vi "test_OneSessTwoPinOneInstrOneSiteReservation_VISAGetConnections1Pin1Connection_ReturnsOneConnection.vi"(8 "error in":errorcluster) -> (0 "error out":errorcluster, 2 "result":string, 3 "pass":bool)   [LabVIEW 2020, in "MeasurementServerTests.lvlib"]
uses:
  MeasurementServerTests.lvlib
  Runtime/MeasurementLink Session Management V1/Session Reservation/Connection.ctl
  Runtime/MeasurementLink VISA/Connection with Session.ctl
  03fc85e1-696b-4ece-a78b-f41470766ac0.vi
  54688eee-c370-47ce-a16a-9847a0fe0368.vi
  <vilib>/AdvancedString/1D String Array to Delimited String.vi
  54688eee-c370-47ce-a16a-9847a0fe0368.vi/94283ac5-2298-4b3a-b57d-7be67da3787d.vi
  54688eee-c370-47ce-a16a-9847a0fe0368.vi/f7d9c9cb-0251-4d67-81cb-70e1b0e8b69f.vi
  Runtime/MeasurementLink VISA/Get Connections - 1Pin 1Conn.vi
  <vilib>/JDP Science/JSONtext/Variant to JSON Text.vi
  <vilib>/JDP Science/JSONtext/LVClass Serializer/JSONtext LVClass Serializer.lvclass
  Runtime/MeasurementLink Session Management V1/Session Reservation/Session Reservation.lvclass
  Runtime/MeasurementLink VISA/MeasurementLink VISA.lvlib
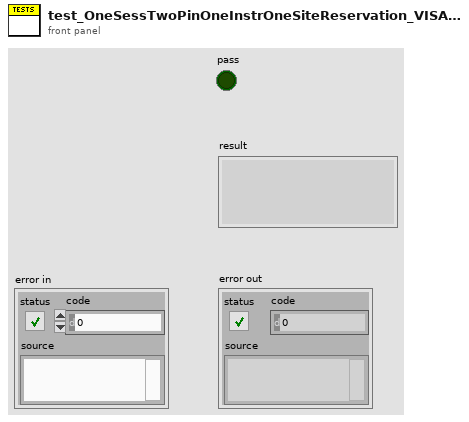
[diagram p1: front panel]
types:
  T1 = typedef "MeasurementLink VISA.lvlib/Connection with Session.ctl" = cluster{"connection":T2, "session":refnum<visa-resource-name>}
  T2 = typedef "MeasurementLink Session Management V1.lvlib/Session Reservation.lvclass/Connection.ctl" = cluster{"pin or relay name":string, "site":i32, "instrument type id":string, "channel":string}
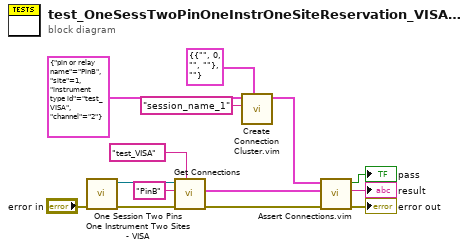
[diagram p0: block diagram]
diagram:
  n1 = call "One Session Two Pins One Instrument Two Sites - VISA.vi"("error in"="error in") -> ("error out"=w4:errorcluster, "session reservation out"=w5:refnum<class "Session Reservation.lvclass">)  [unwired: 9 in]
  n2 = call-poly "Get Connections.vi"("instrument type id"="test_VISA", "error in"=w4, "pin or relay name"="PinB", "session reservation in"=w5) -> ("error out"=w2:errorcluster, "connection"=w14:T1)  [unwired: 5 in, 1 out]
  n3 = call "Create Connection Cluster.vim"("connection type"=T1 {"connection"={"pin or relay name"="", "site"=0, "instrument type id"="", "channel"=""}, "session"=""} ("niDCPower connection"), "session in"="session_name_1", "hardware independent connection in"=T2 {"pin or relay name"="PinB", "site"=1, "instrument type id"="test_VISA", "channel"="2"} ("connection")) -> ("connection out"=w11:T1)  [unwired: 8 in]
  n4 = call "Assert Connections.vim"("error in"=w2, "actual connections"=w14, "expected connections"=w11) -> ("error out"=→"error out":errorcluster, "result"=→"result":string, "pass"=→"pass":bool)  [unwired: 6 in]
